vi "test.Create.ReduceSizeLong.vi"(11 "ReduceSizeLong.Parameters":T1={"Time Offset"=0, "Order Id"="ORID0001", "Canceled Quantity"=200}) -> (3 "Passed":bool)   [LabVIEW 2020]
uses:
  ReduceSize/ReduceSizeLong.Parameters.ctl
  ReduceSize/ReduceSizeLong.lvclass
panel:
  out "x = y?":bool[](array[boolean])
  out "Python.Bytes.Out":u8[](array[numeric]) format="%.0x"
  out "LabVIEW.Bytes.Out":u8[](array[numeric]) format="%.0x"
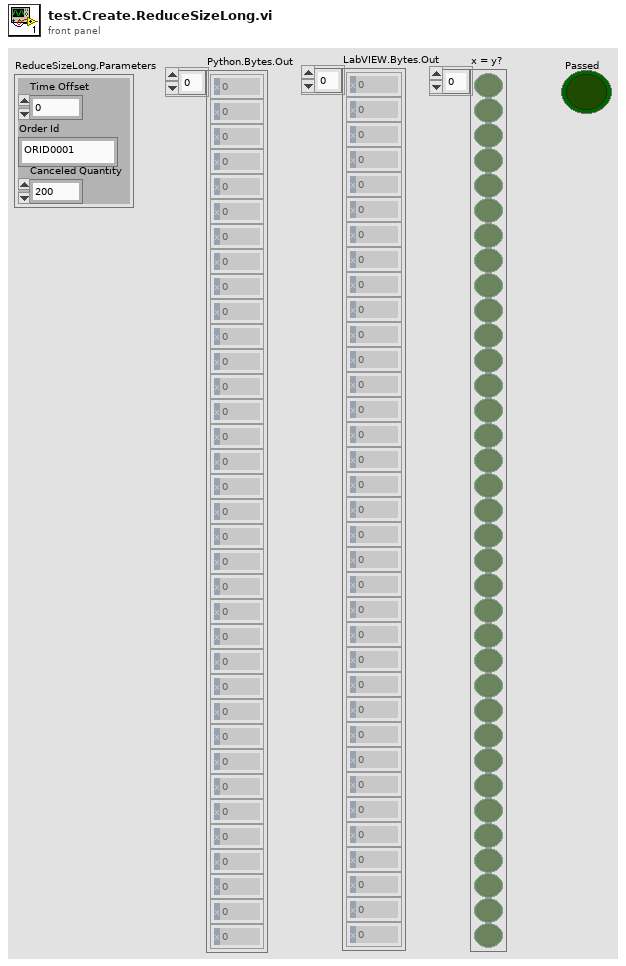
[diagram p1: front panel]
types:
  T1 = typedef "ReduceSizeLong.lvclass/ReduceSizeLong.Parameters.ctl" = cluster{"Time Offset":u32, "Order Id":string, "Canceled Quantity":u32}
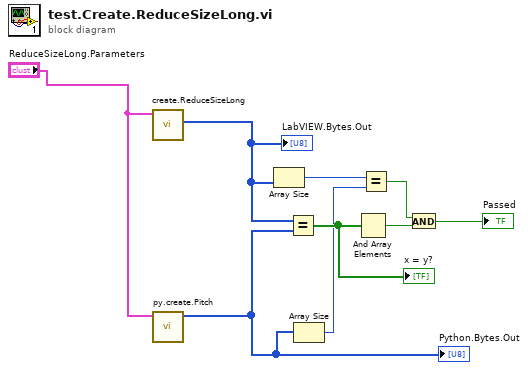
[diagram p0: block diagram]
diagram:
  n1 = call "create.ReduceSizeLong.vi"("ReduceSizeLong.Parameters"="ReduceSizeLong.Parameters") -> ("Bytes.out"=w5:u8[])  [unwired: 8 in, 2 out]
  "LabVIEW.Bytes.Out" <- w5
  n2 = call "py.create.Pitch.vi"("Parameters"="ReduceSizeLong.Parameters") -> ("bytes"=w2:u8[])  [unwired: 9 in, 1 out]
  "Python.Bytes.Out" <- w2
  n3 = Array Size(array=w5) -> (size(s)=w3:i32)
  n4 = Equal?(x=w5, y=w2) -> (x = y?=w9:bool[])
  "x = y?" <- w9
  n5 = Array Size(array=w2) -> (size(s)=w1:i32)
  n6 = And Array Elements(Boolean array=w9) -> (logical AND=w6:bool)
  n7 = Equal?(x=w3, y=w1) -> (x = y?=w4:bool)
  n8 = And(x=w4, y=w6) -> (x .and. y?=→"Passed":bool)
